vi "Source Voltage V3.vi"(8 "error in":errorcluster, 10 "Voltage Level (V)":dbl format="%#_6p", 11 "DCPower SSC in":T1[](array[typedef])) -> (0 "error out":errorcluster, 3 "DCPower SSC out":T1[](array[typedef]))   [LabVIEW 2019]
uses:
  Instrument Control/DCPower/SSC DCPower/SSC DCPower.ctl
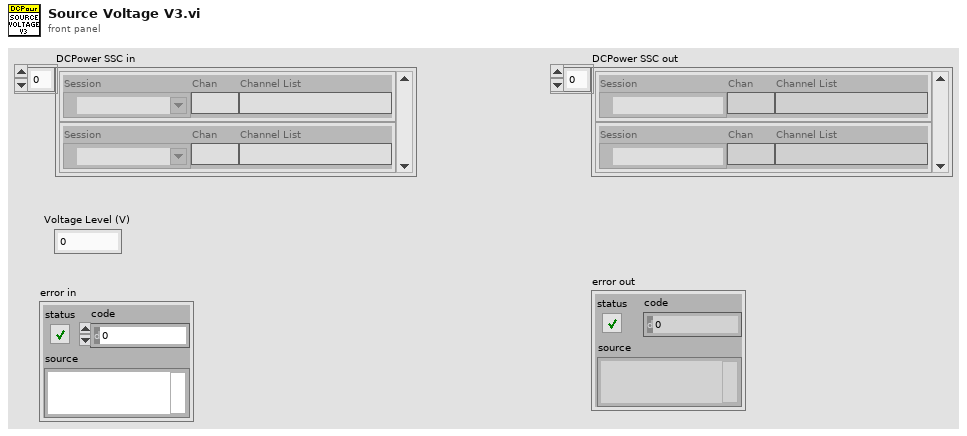
[diagram p1: front panel]
types:
  T1 = typedef "SSC DCPower.ctl" = cluster{"Session":refnum<k15>, "Chan":string, "Channel List":string}
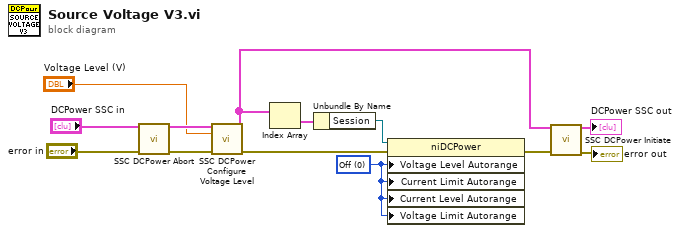
[diagram p0: block diagram]
diagram:
  w1 = 0 items=["Off", "On"] ("Source:DC Voltage:Voltage Level Autorange")
  n1 = call "SSC DCPower Abort.vi"("DCPower SSC in"="DCPower SSC in", "error in"="error in") -> ("DCPower SSC out"=w13:T1[], "error out"=w12:errorcluster)  [unwired: 12 in]
  n2 = call "SSC DCPower Configure Voltage Level.vi"("DCPower SSC in"=w13, "Voltage Level (V)"="Voltage Level (V)", "error in"=w12) -> ("DCPower SSC out"=w4:T1[], "error out"=w6:errorcluster)  [unwired: 11 in]
  n3 = Index Array(array=w4) -> (element=w3:T1)  [unwired: 1 in]
  n4 = Unbundle By Name(w3) -> ("Session"=w2:refnum<k15>)
  n5 = property class="niDCPower"(reference=w2, error in=w6, "Voltage Level Autorange"=w1, "Current Limit Autorange"=w1, "Current Level Autorange"=w1, "Voltage Limit Autorange"=w1) -> (error out=w5:errorcluster)  [unwired: 1 out]
  n6 = call "SSC DCPower Initiate.vi"("DCPower SSC in"=w4, "error in"=w5) -> ("DCPower SSC out"=→"DCPower SSC out":T1[], "error out"=→"error out":errorcluster)  [unwired: 12 in]
